vi "Connect.vi"(8 "error in (no error)":errorcluster, 10 "Serial Config":T1={"Baud"=9600, "Flow Ctl"=0, "Parity"=0, "COM Port"="COM3", "Address"=1} {"Parity" items=["None", "Odd", "Even"]; "Flow Ctl" items=["None"]; "Baud" items=["4800"=4800, "9600"=9600, "19200"=19200, "38400"=38400]}, 11 "Omega CN9600 series.lvclass":refnum<class "Omega CN9600 series.lvclass">) -> (0 "error out":errorcluster, 3 "Omega CN9600 series.lvclass 2":refnum<class "Omega CN9600 series.lvclass">)   [LabVIEW 2014, in "Omega CN9600 series.lvclass"]
uses:
  Omega CN9600 series.lvclass
  Serial_Config_Omega.ctl
  Omega CN9600 series.lvclass/Omega CN9600 series.ctl
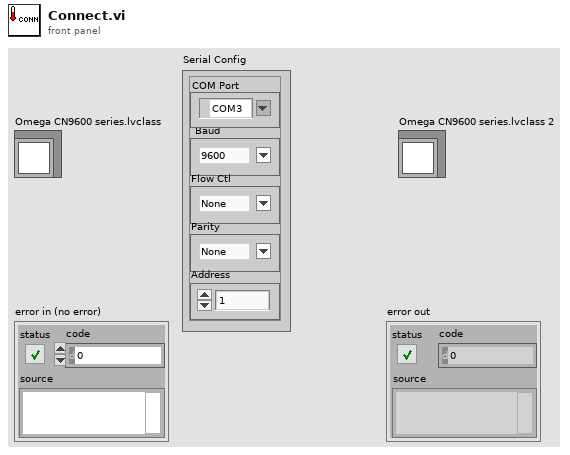
[diagram p1: front panel]
types:
  T1 = typedef "Omega CN9600 series.lvclass/Serial_Config_Omega.ctl" = cluster{"Baud":u32, "Flow Ctl":u16, "Parity":u16, "COM Port":refnum<visa-resource-name>, "Address":u8}
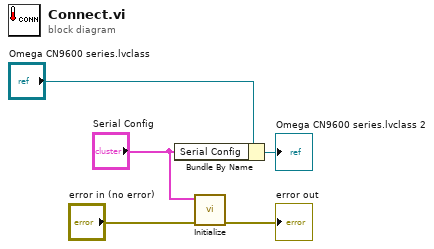
[diagram p0: block diagram]
diagram:
  n1 = Bundle By Name(cluster="Omega CN9600 series.lvclass", "Serial Config"="Serial Config") -> (→"Omega CN9600 series.lvclass 2":refnum<class "Omega CN9600 series.lvclass">)
  n2 = call "Initialize.vi"("error in (no error)"="error in (no error)", "Serial Config"="Serial Config") -> ("error out"=→"error out":errorcluster)  [unwired: 8 in, 1 out]
